vi "Set Version String.vi"(8 "error in (no error)":errorcluster, 9 "Version String":string, 10 "App":refnum<vi>) -> (0 "error out":errorcluster)   [LabVIEW 2020, in "VolatusBuild.lvlib"]
uses:
  VolatusBuild.lvlib
  <vilib>/Utility/traverseref.llb/TRef TravTarget.ctl
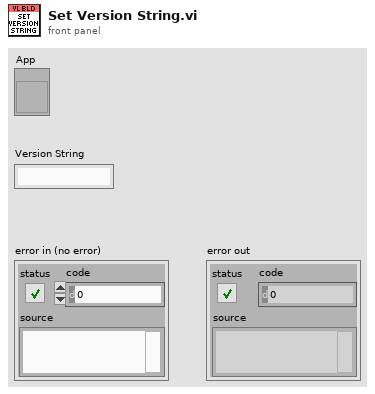
[diagram p1: front panel]
types:
  T1 = typedef "TRef TravTarget.ctl" = enum16{"FP", "BD", "Other"}
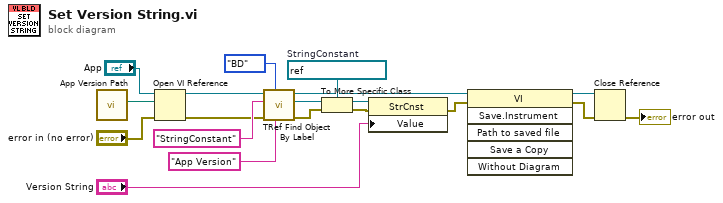
[diagram p0: block diagram]
diagram:
  w14 = refnum<vi> refnum  # StringConstant
  n1 = call "App Version Path.vi"() -> ("App Version.vi"=w5:path)  [unwired: 11 in]
  n2 = Open VI Reference(application reference (local)="App", vi path=w5, error in (no error)="error in (no error)") -> (vi reference=w19:refnum<vi>, error out=w4:errorcluster)  [unwired: 3 in]
  n3 = call <vilib>:"TRef Find Object By Label.vi"("Label"="App Version" ("Class Name"), "Traverse Target"=TRef_TravTarget."BD", "error in (no error)"=w4, "Class Name"="StringConstant", "VI Ref"=w19) -> ("error out"=w13:errorcluster, "Found Obj Ref"=w15:refnum<vi>, "dup VI Ref"=w10:refnum<vi>)  [unwired: 3 in, 1 out]
  n4 = To More Specific Class(target class=w14, reference=w15, error in=w13) -> (specific class reference=w12:refnum<vi>, error out=w11:errorcluster)
  n5 = property class="StrCnst"(reference=w12, error in=w11, "Value"="Version String") -> (error out=w9:errorcluster)  [unwired: 1 out]
  n6 = invoke class="VI" method="Save.Instrument"(reference=w10, error in=w9) -> (reference out=w8:refnum<vi>, error out=w7:errorcluster)  [unwired: 4 in, 4 out]
  n7 = Close Reference(reference=w8, error in (no error)=w7) -> (error out=→"error out":errorcluster)
